vi "PSTRA-Export Raw Data File.vi"(0 "Path":path, 7 "Runtime in":T1 {"window" items=["None ", "Hanning", "Hamming", "Blackman-Harris", "Exact Blackman", "Blackman", "Flat Top", "4 Term B-Harris ", "7 Term B-Harris", "Low Sidelobe"]}, 11 "error in (no error)":errorcluster) -> (15 "error out":errorcluster)   [LabVIEW 2020]
uses:
  <userlib>/_matio/level5/Public/Write/Append Data Element.llb/Append Data Element (1D Array of Double).vi
  Typedefs/PSTR-Runtime Data.ctl
  epl-vi-lib/Signal Synthesis VIs/4th Generation/Classes/SignalManager/SignalManager.lvclass
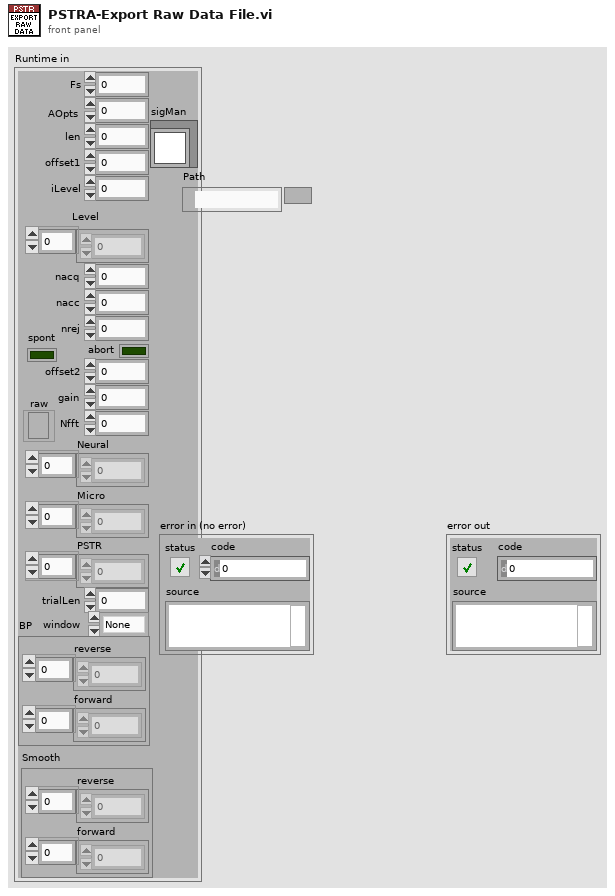
[diagram p1: front panel]
types:
  T1 = typedef "PSTR-Runtime Data.ctl" = cluster{"Fs":dbl, "AOpts":i32, "len":i32, "offset1":i32, "iLevel":i32, "Level":dbl[], "nacc":i32, "nrej":i32, "nacq":i32, "abort":bool, "offset2":i32, "gain":dbl, "Nfft":i32, "Neural":dbl[], "Micro":dbl[], "raw":refnum<file>, "spont":bool, "PSTR":dbl[], "trialLen":i32, "window":u16, "BP":cluster{"reverse":dbl[], "forward":dbl[]}, "Smooth":cluster{"reverse":dbl[], "forward":dbl[]}, "sigMan":refnum<class "SignalManager.lvclass">}
  T2 = enum16{"big-endian, network order", "native, host order", "little-endian"}
  T3 = enum16{"open", "replace", "create", "open or create", "replace or create", "replace or create with confirmation"}
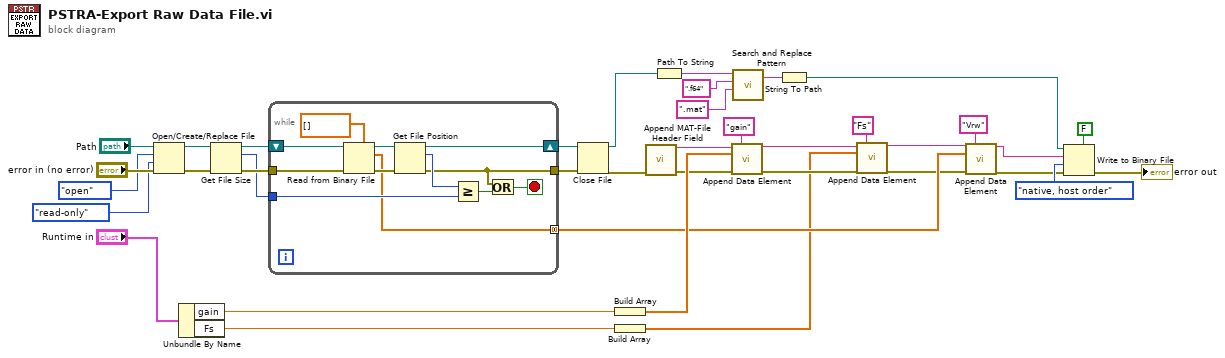
[diagram p0: block diagram]
diagram:
  n1 = Open/Create/Replace File(file path (use dialog)="Path", error in="error in (no error)", operation (0:open)=T3."open", access (0:read/write)=enum16{"read/write", "read-only", "write-only"}."read-only") -> (refnum out=w33:refnum<file>, error out=w28:errorcluster)  [unwired: 2 in, 1 out]
  n2 = Unbundle By Name("Runtime in") -> ("gain"=w16:dbl, "Fs"=w8:dbl)
  n3 = Get File Size(file=w33, error in=w28) -> (refnum out=w30:refnum<file>, size (in bytes)=w27:i64, 0:w29:errorcluster)
  n4 = while {
    tunnel: w29 -> [w47]
    shift-right: [w45] -> w32
    shift-left: w30 -> [w49]
    tunnel: [w41] -> w31
    tunnel: w27 -> [w43]
    tunnel: [w39] -> w15 mode=concatenating
    stop <- w40 stop-if-true
    n5 = Read from Binary File(5:dbl[] [] ("data"), 8:w47, 11:w49) -> (0:w41:errorcluster, 2:w39:dbl[], 3:w46:refnum<file>)  [unwired: 3 in, 1 out]
    n6 = Get File Position(7:w46) -> (2:w44:i64, 3:w45:refnum<file>)  [unwired: 1 in, 1 out]
    n7 = Greater Or Equal?(x=w44, y=w43) -> (x >= y?=w42:bool)
    n8 = Or(x=w41, y=w42) -> (x .or. y?=w40:bool)
  }
  n9 = Close File(refnum=w32, error in=w31) -> (path=w6:path, error out=w17:errorcluster)
  n10 = Build Array(w16) -> (w26:dbl[])
  n11 = Build Array(w8) -> (w7:dbl[])
  n12 = call <userlib>:"Append MAT-File Header Field.vi"("error"=w17) -> ("result string"=w23:string, "error out"=w24:errorcluster)  [unwired: 13 in]
  n13 = Path To String(path=w6) -> (string=w5:string)
  n14 = call-poly <userlib>:"Append Data Element.vi"("initial string"=w23, "Data Name"="gain", "data"=w26, "error in"=w24) -> ("result string"=w12:string, "error out"=w13:errorcluster)  [unwired: 10 in]
  n15 = call <vilib>:"Search and Replace Pattern.vi"("string"=w5, "regular expression (\"\")"=".f64" ("regular expression (\"\")"), "replace string (\"\")"=".mat" ("regular expression (\"\")")) -> ("result string"=w2:string)  [unwired: 2 in, 1 out]
  n16 = String To Path(string=w2) -> (path=w1:path)
  n17 = call-poly <userlib>:"Append Data Element.vi"("initial string"=w12, "Data Name"="Fs", "data"=w7, "error in"=w13) -> ("result string"=w11:string, "error out"=w10:errorcluster)  [unwired: 10 in]
  n18 = call-poly <userlib>:"Append Data Element.vi"("initial string"=w11, "Data Name"="Vrw", "data"=w15, "error in"=w10) -> ("result string"=w20:string, "error out"=w19:errorcluster)  [unwired: 10 in]
  n19 = Write to Binary File(file (use dialog)=w1, data=w20, error in=w19, 5:FALSE ("prepend array or string size? (T)"), 9:T2."native, host order" ("byte order (0:big-endian, network order)")) -> (error out=→"error out":errorcluster)  [unwired: 1 in, 2 out]
